vi "SSFG_simulated.vi"() -> ()   [LabVIEW 2014]
uses:
  SSFG_States.ctl
  <vilib>/Utility/error.llb/DialogType.ctl
  <vilib>/DAQmx/write.llb/DAQmx Write (Analog Wfm 1Chan NSamp).vi
  <vilib>/DAQmx/create/channels.llb/DAQmx Create Channel (AO-Voltage-Basic).vi
  <vilib>/DAQmx/configure/timing.llb/DAQmx Timing (Sample Clock).vi
  <vilib>/DAQmx/miscellaneous.llb/DAQmx Fill In Error Info.vi
  <resource>/objmgr/daqmx.rc
  <vilib>/measure/NI_MABase.lvlib
panel:
  in  "#s":dbl
  out "Waveform Graph":waveform(dbl)(graph)
  in  "stop":bool
  in  "Power Signal Parameters":T1={"Waveform Type"=0, "Amplitude"=1.0, "Frequency"=17.0} {"Frequency" format="%0.2p"; "Amplitude" scale=0.0..5.0; "Waveform Type" items=["Sine Wave", "Triangle Wave", "Square Wave", "Sawtooth Wave"]}
  out "Flicker":bool
  out "Swell":bool
  out "Sag":bool
  in  "Stop":bool
  in  "Update Rate":dbl=1000.0 format="%0.2f"
  in  "Physical Channel":tag
  in  "Flicker":T2
  in  "Swell":cluster{"Swell_Time (sec)":dbl, "Swell":bool}
  in  "Sag":cluster{"Sag_Time (sec)":dbl, "Sag":bool}
  in  "Power Signal":bool
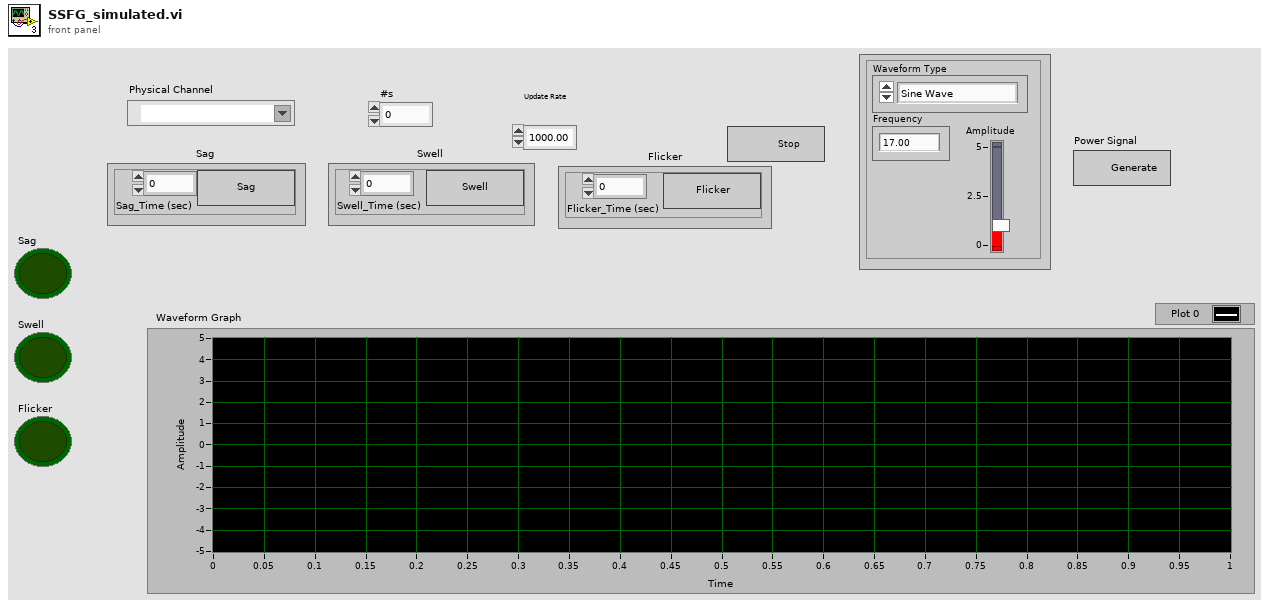
[diagram p1: front panel]
types:
  T1 = cluster{"Waveform Type":u16, "Amplitude":dbl, "Frequency":dbl}
  T2 = cluster{"Flicker_Time (sec)":dbl, "Flicker":bool}
  T3 = typedef "DialogType.ctl" = u16
  T4 = typedef "SSFG_States.ctl" = cluster{"State":string, "Disturbance_Time (sec)":dbl}
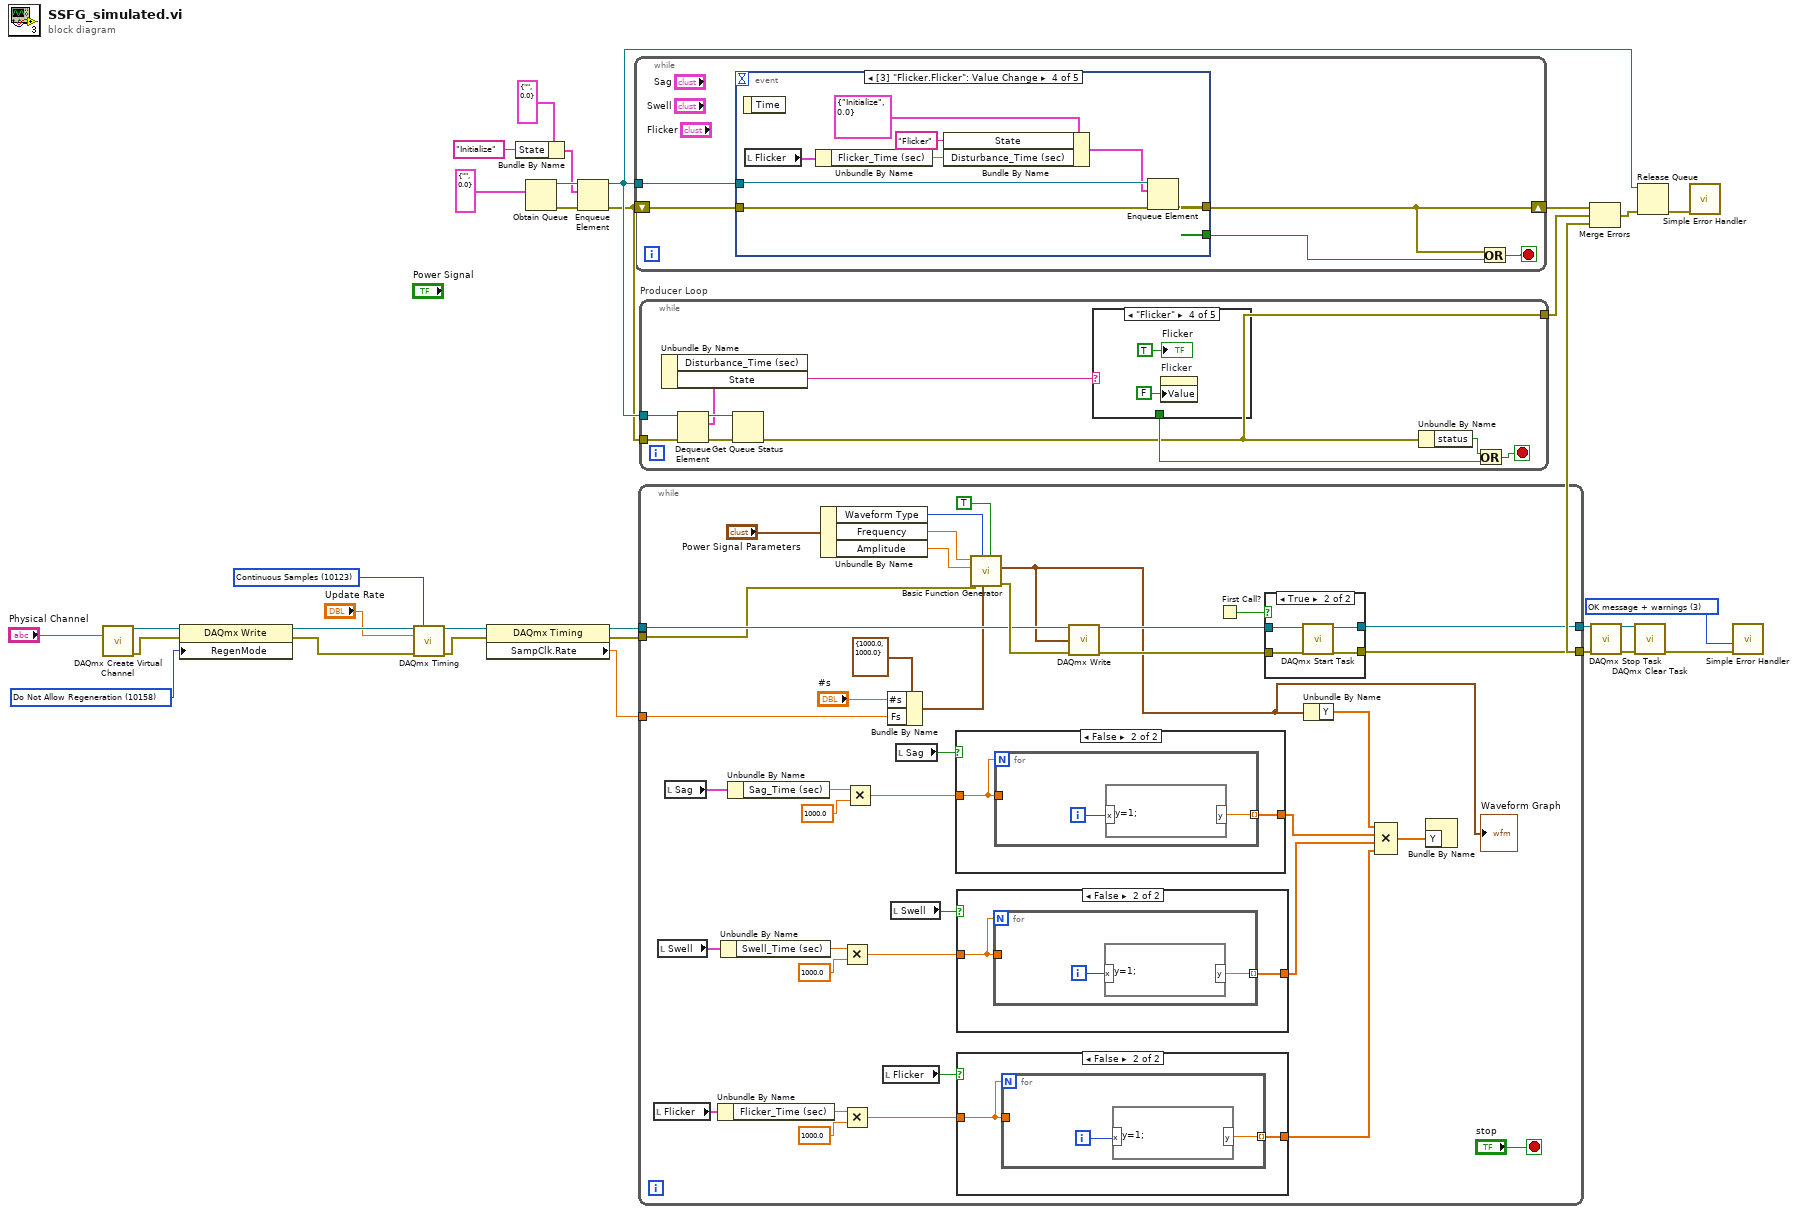
[diagram p0: block diagram]
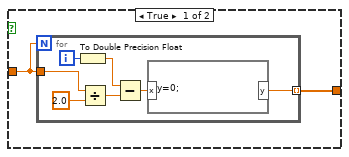
[diagram p2: hidden frame]
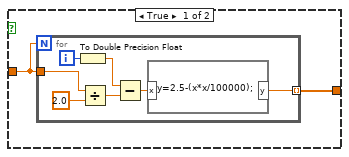
[diagram p3: hidden frame]
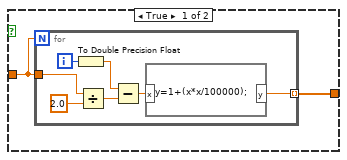
[diagram p4: hidden frame]
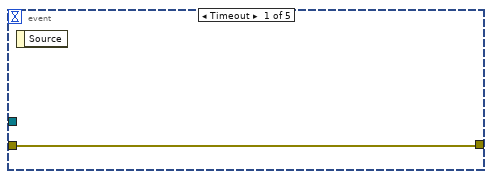
[diagram p6: hidden frame]
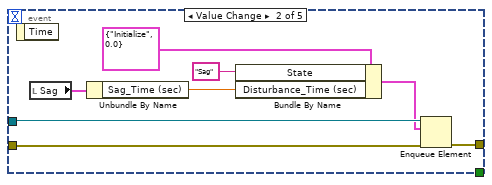
[diagram p7: hidden frame]
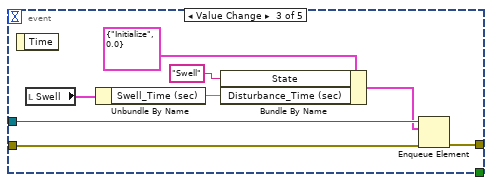
[diagram p8: hidden frame]
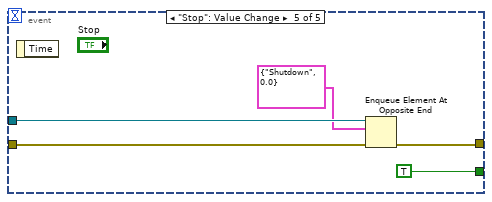
[diagram p9: hidden frame]
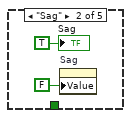
[diagram p11: hidden frame]
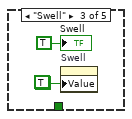
[diagram p12: hidden frame]
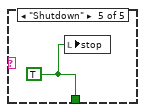
[diagram p13: hidden frame]
diagram:
  w6 = T3 3 items=["no dialog", "OK message", "continue or stop message", "OK message + warnings", "continue/stop + warnings"] ("type of dialog (OK msg:1)")
  w25 = 10123 items=["Finite Samples"=10178, "Continuous Samples"=10123, "Hardware Timed Single Point"=12522] ("sample mode")
  w26 = 10158 items=["Allow Regeneration"=10097, "Do Not Allow Regeneration"=10158] ("RegenMode")
  n1 = call-poly <vilib>:"DAQmx Create Virtual Channel.vi"("physical channels"="Physical Channel") -> ("task out"=w30:refnum<k21>, "error out"=w28:errorcluster)  [unwired: 13 in]
  n2 = property class="DAQmx Write"(reference=w30, error in=w28, "RegenMode"=w26) -> (reference out=w29:refnum<k21>, error out=w27:errorcluster)
  n3 = call-poly <vilib>:"DAQmx Timing.vi"("task/channels in"=w29, "sample mode"=w25, "rate"="Update Rate", "error in"=w27) -> ("task out"=w23:refnum<k21>, "error out"=w22:errorcluster)  [unwired: 10 in]
  n4 = property class="DAQmx Timing"(reference=w23, error in=w22) -> (reference out=w3:refnum<k21>, error out=w4:errorcluster, "SampClk.Rate"=w2:dbl)
  n5 = Bundle By Name(cluster=T4 {"State"="", "Disturbance_Time (sec)"=0.0}, "State"="Initialize") -> (w14:T4)
  n6 = Obtain Queue(element data type=T4 {"State"="", "Disturbance_Time (sec)"=0.0}) -> (queue out=w18:refnum<queue>, error out=w17:errorcluster)  [unwired: 4 in, 1 out]
  n7 = Enqueue Element(queue=w18, element=w14, error in (no error)=w17) -> (queue out=w12:refnum<queue>, error out=w11:errorcluster)  [unwired: 1 in, 1 out]
  n8 = while {
    tunnel: w12 -> [w35]
    shift-right: [w33] -> w20
    shift-left: w11 -> [w34]
    stop <- w36 stop-if-true
    n9 = event shown="[3] \"Flicker.Flicker\": Value Change" {
      selector: _ -> [_ _ _ _ _]
      dyn-events: _ -> [_ _ _ _ _]
      timeout: _ -> [_ _ _ _ _]
      tunnel: w35 -> [_ w45 w53 w61 w66]
      tunnel: w34 -> [w37 w44 w52 w60 w65]
      tunnel: [w37 w43 w51 w59 w64] -> w33
      tunnel: [_ _ _ _ TRUE] -> w32
      event Timeout {
        n10 = event-data() -> ()  [unwired: 1 in, 1 out]
      }
      event "Sag.Sag": Value Change {
        n11 = event-data() -> ()  [unwired: 1 in, 1 out]
        n12 = local read "Sag"() -> (w38:cluster{"Sag_Time (sec)":dbl, "Sag":bool})
        n13 = Unbundle By Name(w38) -> ("Sag_Time (sec)"=w40:dbl)
        n14 = Bundle By Name(cluster=T4 {"State"="Initialize", "Disturbance_Time (sec)"=0.0}, "State"="Sag", "Disturbance_Time (sec)"=w40) -> (w39:T4)
        n15 = Enqueue Element(queue=w45, element=w39, error in (no error)=w44) -> (error out=w43:errorcluster)  [unwired: 1 in, 2 out]
      }
      event "Swell.Swell": Value Change {
        n16 = event-data() -> ()  [unwired: 1 in, 1 out]
        n17 = local read "Swell"() -> (w46:cluster{"Swell_Time (sec)":dbl, "Swell":bool})
        n18 = Unbundle By Name(w46) -> ("Swell_Time (sec)"=w49:dbl)
        n19 = Bundle By Name(cluster=T4 {"State"="Initialize", "Disturbance_Time (sec)"=0.0}, "State"="Swell", "Disturbance_Time (sec)"=w49) -> (w47:T4)
        n20 = Enqueue Element(queue=w53, element=w47, error in (no error)=w52) -> (error out=w51:errorcluster)  [unwired: 1 in, 2 out]
      }
      event "Flicker.Flicker": Value Change {
        n21 = event-data() -> ()  [unwired: 1 in, 1 out]
        n22 = local read "Flicker"() -> (w54:T2)
        n23 = Unbundle By Name(w54) -> ("Flicker_Time (sec)"=w56:dbl)
        n24 = Bundle By Name(cluster=T4 {"State"="Initialize", "Disturbance_Time (sec)"=0.0}, "State"="Flicker", "Disturbance_Time (sec)"=w56) -> (w55:T4)
        n25 = Enqueue Element(queue=w61, element=w55, error in (no error)=w60) -> (error out=w59:errorcluster)  [unwired: 1 in, 2 out]
      }
      event "Stop": Value Change {
        n26 = event-data() -> ()  [unwired: 1 in, 1 out]
        n27 = Enqueue Element At Opposite End(queue=w66, element=T4 {"State"="Shutdown", "Disturbance_Time (sec)"=0.0}, error in (no error)=w65) -> (error out=w64:errorcluster)  [unwired: 1 in, 2 out]
      }
    }
    n28 = Or(x=w33, y=w32) -> (x .or. y?=w36:bool)
  }
  n29 = while {
    tunnel: [w95] -> w1
    tunnel: [w94] -> w5
    tunnel: w3 -> [w93]
    tunnel: w4 -> [w92]
    tunnel: w2 -> [w69]
    stop <- "stop" stop-if-true
    n30 = local read "Flicker"() -> (w75:T2)
    n31 = local read "Swell"() -> (w78:cluster{"Swell_Time (sec)":dbl, "Swell":bool})
    n32 = local read "Sag"() -> (w81:cluster{"Sag_Time (sec)":dbl, "Sag":bool})
    n33 = Unbundle By Name(w75) -> ("Flicker_Time (sec)"=w73:dbl)
    n34 = Unbundle By Name(w78) -> ("Swell_Time (sec)"=w76:dbl)
    n35 = Unbundle By Name(w81) -> ("Sag_Time (sec)"=w79:dbl)
    n36 = Unbundle By Name("Power Signal Parameters") -> ("Waveform Type"=w100:u16, "Frequency"=w99:dbl, "Amplitude"=w98:dbl)
    n37 = Multiply(x=w76, y=1000.0) -> (x*y=w71:dbl)
    n38 = Multiply(x=w73, y=1000.0) -> (x*y=w70:dbl)
    n39 = Multiply(x=w79, y=1000.0) -> (x*y=w72:dbl)
    n40 = local read "Flicker"() -> (w83:bool)
    n41 = Bundle By Name(cluster=cluster{"Fs":dbl, "#s":dbl} {"Fs"=1000.0, "#s"=1000.0} ("sampling info"), "#s"="#s", "Fs"=w69) -> (w90:cluster{"Fs":dbl, "#s":dbl})
    n42 = local read "Swell"() -> (w89:bool)
    n43 = local read "Sag"() -> (w91:bool)
    n44 = case shown="False" w91 {
      tunnel: [w133 w142] -> w88
      tunnel: w72 -> [w132 w141]
      frame True {
        n45 = for {
          N: w132 -> [_]
          tunnel: w132 -> [w139]
          tunnel: [w134] -> w133 mode=indexing
          i -> [w136]
          n46 = To Double Precision Float(number=w136) -> (double precision float=w137:dbl)
          n47 = Divide(x=w139, y=2.0) -> (x/y=w138:dbl)
          n48 = Subtract(x=w137, y=w138) -> (x-y=w135:dbl)
          n49 = formula code="y=1+(x*x/100000);"("x"=w135) -> ("y"=w134:dbl)
        }
      }
      frame False {
        n50 = for {
          N: w141 -> [_]
          tunnel: w141 -> [_]
          tunnel: [w144] -> w142 mode=indexing
          i -> [w143]
          n51 = formula code="y=1;"("x"=w143) -> ("y"=w144:dbl)
        }
      }
    }
    n52 = case shown="False" w89 {
      tunnel: [w120 w129] -> w87
      tunnel: w71 -> [w119 w128]
      frame True {
        n53 = for {
          N: w119 -> [_]
          tunnel: w119 -> [w126]
          tunnel: [w121] -> w120 mode=indexing
          i -> [w123]
          n54 = To Double Precision Float(number=w123) -> (double precision float=w124:dbl)
          n55 = Divide(x=w126, y=2.0) -> (x/y=w125:dbl)
          n56 = Subtract(x=w124, y=w125) -> (x-y=w122:dbl)
          n57 = formula code="y=2.5-(x*x/100000);"("x"=w122) -> ("y"=w121:dbl)
        }
      }
      frame False {
        n58 = for {
          N: w128 -> [_]
          tunnel: w128 -> [_]
          tunnel: [w131] -> w129 mode=indexing
          i -> [w130]
          n59 = formula code="y=1;"("x"=w130) -> ("y"=w131:dbl)
        }
      }
    }
    n60 = case shown="False" w83 {
      tunnel: [w107 w116] -> w86
      tunnel: w70 -> [w106 w115]
      frame True {
        n61 = for {
          N: w106 -> [_]
          tunnel: w106 -> [w113]
          tunnel: [w108] -> w107 mode=indexing
          i -> [w110]
          n62 = To Double Precision Float(number=w110) -> (double precision float=w111:dbl)
          n63 = Divide(x=w113, y=2.0) -> (x/y=w112:dbl)
          n64 = Subtract(x=w111, y=w112) -> (x-y=w109:dbl)
          n65 = formula code="y=0;"("x"=w109) -> ("y"=w108:dbl)
        }
      }
      frame False {
        n66 = for {
          N: w115 -> [_]
          tunnel: w115 -> [_]
          tunnel: [w118] -> w116 mode=indexing
          i -> [w117]
          n67 = formula code="y=1;"("x"=w117) -> ("y"=w118:dbl)
        }
      }
    }
    n68 = call <vilib>:"Basic Function Generator.vi"("reset signal"=TRUE, "sampling info"=w90, "signal type"=w100, "error in (no error)"=w92, "amplitude"=w98, "frequency"=w99) -> ("error out"=w102:errorcluster, "signal out"=w68:waveform(dbl))  [unwired: 3 in, 1 out]
    "Waveform Graph" <- w68
    n69 = call-poly <vilib>:"DAQmx Write.vi"("task/channels in"=w93, "data"=w68, "error in"=w102) -> ("task out"=w104:refnum<k21>, "error out"=w103:errorcluster)  [unwired: 10 in, 1 out]
    n70 = First Call?() -> (First Call?: T/F=w101:bool)
    n71 = case shown="True" w101 {
      tunnel: w104 -> [w145 w150]
      tunnel: w103 -> [w146 w149]
      tunnel: [w145 w148] -> w94
      tunnel: [w146 w147] -> w95
      frame False {
      }
      frame True {
        n72 = call <vilib>:"DAQmx Start Task.vi"("task/channels in"=w150, "error in"=w149) -> ("task out"=w148:refnum<k21>, "error out"=w147:errorcluster)  [unwired: 12 in]
      }
    }
    n73 = Unbundle By Name(w68) -> ("Y"=w85:dbl[])
    n74 = Compound Arithmetic op=MULTIPLY(w85, w88, w87, w86) -> (w84:dbl[])
    n75 = Bundle By Name("Y"=w84) -> ()  [unwired: 1 in, 1 out]
  }
  n76 = while "Producer Loop" {
    tunnel: [w151] -> w10
    tunnel: w12 -> [w156]
    tunnel: w11 -> [w155]
    stop <- w160 stop-if-true
    n77 = Dequeue Element(queue=w156, error in (no error)=w155) -> (queue out=w158:refnum<queue>, element=w154:T4, error out=w157:errorcluster)  [unwired: 1 in, 1 out]
    n78 = Unbundle By Name(w154) -> ("State"=w153:string)  [unwired: 1 out]
    n79 = Get Queue Status(queue=w158, error in (no error)=w157) -> (error out=w151:errorcluster)  [unwired: 1 in, 7 out]
    n80 = case shown="\"Flicker\"" w153 {
      tunnel: [_ _ _ _ w167] -> w152
      frame Default {
      }
      frame "Sag" {
        n81 = property on="Sag" class="Bool (strict)"("Value"=FALSE ("Sag")) -> ()  [unwired: 2 in, 2 out]
        "Sag" <- TRUE ("Sag")
      }
      frame "Swell" {
        (unwired) TRUE ("Swell")
        n82 = property on="Swell" class="Bool (strict)"("Value"=FALSE ("Swell")) -> ()  [unwired: 2 in, 2 out]
        "Swell" <- TRUE ("Swell")
      }
      frame "Flicker" {
        n83 = property on="Flicker" class="Bool (strict)"("Value"=FALSE) -> ()  [unwired: 2 in, 2 out]
        "Flicker" <- TRUE ("Flicker")
      }
      frame "Shutdown" {
        w167 = TRUE
        n84 = local write "stop"(w167) -> ()
      }
    }
    n85 = Unbundle By Name(w151) -> ("status"=w159:bool)
    n86 = Or(x=w159, y=w152) -> (x .or. y?=w160:bool)
  }
  n87 = Merge Errors(w20, w10, w1) -> (w19:errorcluster)
  n88 = call <vilib>:"DAQmx Stop Task.vi"("task/channels in"=w5, "error in"=w1) -> ("task out"=w8:refnum<k21>, "error out"=w7:errorcluster)  [unwired: 12 in]
  n89 = call <vilib>:"DAQmx Clear Task.vi"("task in"=w8, "error in"=w7) -> ("error out"=w9:errorcluster)  [unwired: 13 in]
  n90 = Release Queue(queue=w12, error in (no error)=w19) -> (error out=w21:errorcluster)  [unwired: 1 in, 2 out]
  n91 = call <vilib>:"Simple Error Handler.vi"("error in (no error)"=w21) -> ()  [unwired: 4 in, 5 out]
  n92 = call <vilib>:"Simple Error Handler.vi"("type of dialog (OK msg:1)"=w6, "error in (no error)"=w9) -> ()  [unwired: 3 in, 5 out]
